vi "RAMP_save_Z_scan_positions.vi"(2 "error in":errorcluster, 3 "base path":path, 4 "Z array":dbl[](array[numeric])) -> (0 "error out":errorcluster)   [LabVIEW 2015]
uses:
  <vilib>/Utility/file.llb/Write Delimited Spreadsheet (DBL).vi
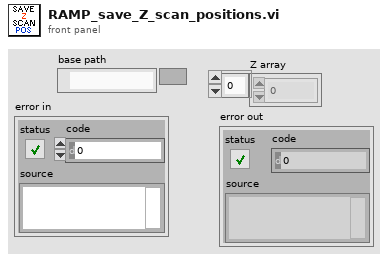
[diagram p1: front panel]
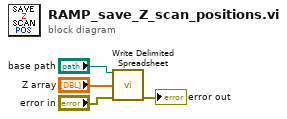
[diagram p0: block diagram]
diagram:
  n1 = call-poly <vilib>:"Write Delimited Spreadsheet.vi"("file path (dialog if empty)"="base path", "1D data"="Z array", "error in (no error)"="error in") -> ("error out"=→"error out":errorcluster)  [unwired: 11 in, 1 out]
